vi "ADC_WRITE CONFIG.vi"(7 "Espera acceso USB":u32, 8 "error in 2":errorcluster, 10 "Dac Data IN":u16, 11 "ftHandle_in 2":u32) -> (0 "error out":errorcluster, 3 "ftHandle_out":u32)   [LabVIEW 2019]
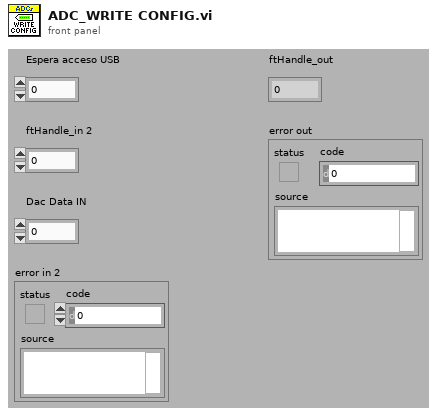
[diagram p1: front panel]
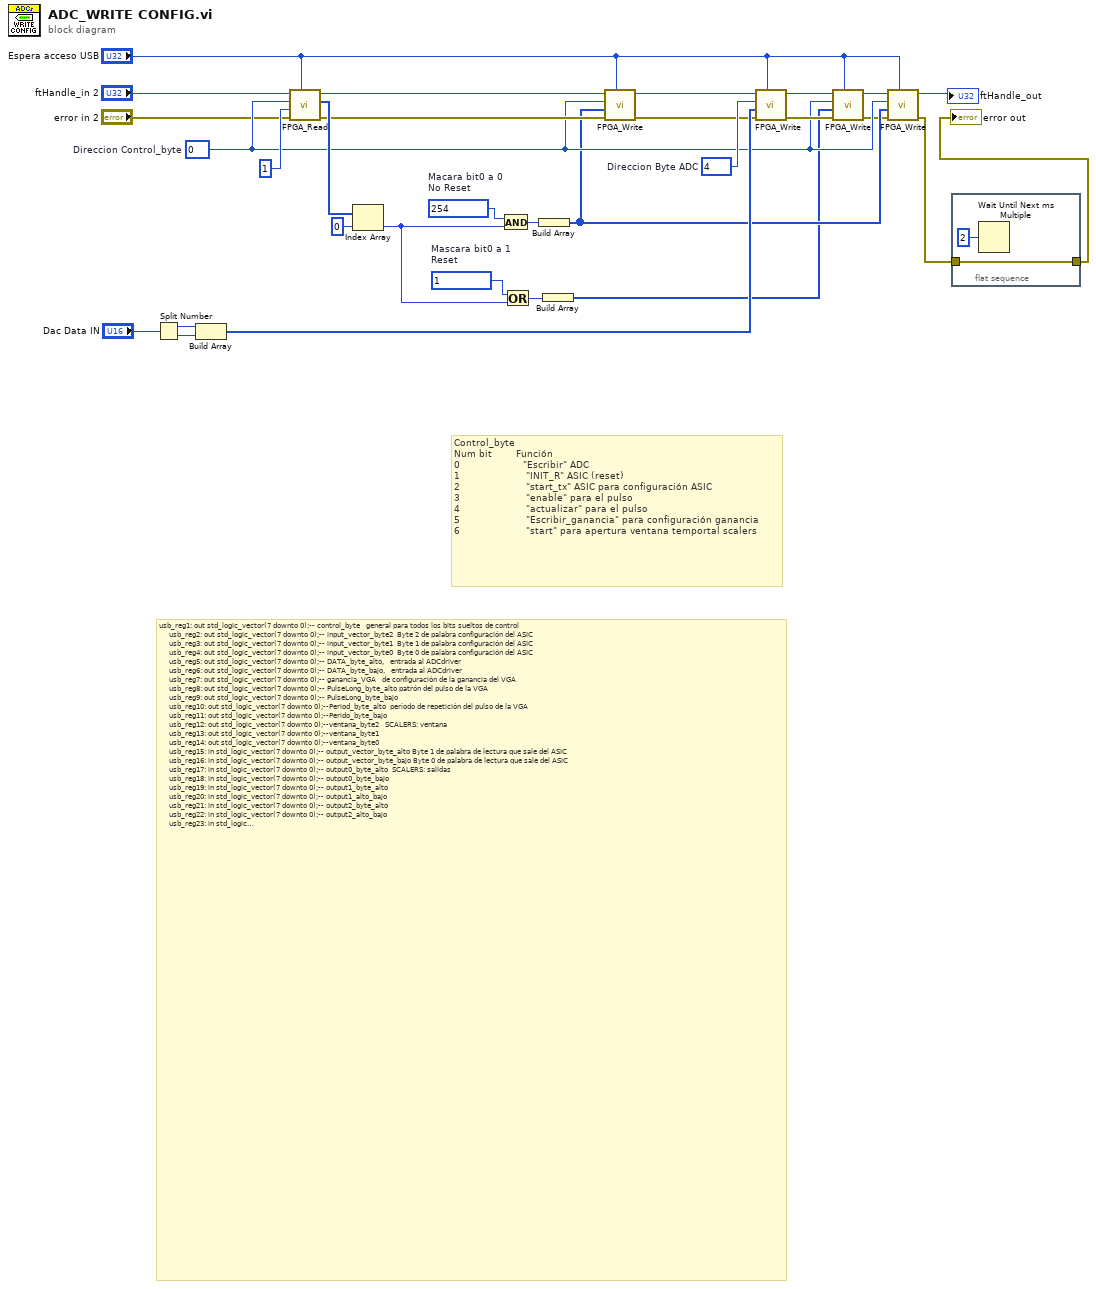
[diagram p0: block diagram]
diagram:
  w26 = u8 4  # Direccion Byte ADC
  w20 = u8 1  # Mascara bit0 a 1 Reset
  w18 = u8 254  # Macara bit0 a 0 No Reset
  w10 = u8 0  # Direccion Control_byte
  # "Control_byte\nNum bit        Función\n0                     \"Escribir\" ADC\n1                      \"INIT_R\" ASIC (reset)\n2                      \"start_tx\" ASIC para configuración ASIC\n3                      \"enable\" para el pulso\n4                      \"actualizar\" para el pulso\n5                      \"Escribir_ganancia\" para configuración ganancia\n6                      \"start\" para apertura ventana temportal scalers"
  # "usb_reg1: out std_logic_vector(7 downto 0);-- control_byte\t\t\tgeneral para todos los bits sueltos de control\n\t\t\t  usb_reg2: out std_logic_vector(7 downto 0);-- input_vector_byte2 \tByte 2 de palabra configuración del ASIC\n\t\t\t  usb_reg3: out std_logic_vector(7 downto 0);-- input_vector_byte1 \tByte 1 de palabra configuración del ASIC\n\t\t\t  usb_reg4: out std_logic_vector(7 downto 0);-- input_vector_byte0 \tByte 0 de palabra configuración del ASIC\n\t\t\t  usb_reg5: out std_logic_vector(7 downto 0);-- DATA_byte_alto, \t\tentrada al ADCdriver\n\t\t\t  usb_reg6: out std_logic_vector(7 downto 0);-- DATA_byte_bajo, \t\tentrada al ADCdriver\n\t\t\t  usb_reg7: out std_logic_vector(7 downto 0);-- ganancia_VGA\t\t\tde configuración de la ganancia del VGA\n\t\t\t  usb_reg8: out std_logic_vector(7 downto 0);-- PulseLong_byte_alto\tpatrón del pulso de la VGA\n\t\t\t  usb_reg9: out std_logic_vector(7 downto 0);-- PulseLong_byte_bajo\n\t\t\t  usb_reg10: out std_logic_vector(7 downto 0);--Period_byte_alto\t\tperíodo de repetición del pulso de la VGA\n\t\t\t  usb_reg11: out std_logic_vector(7 downto 0);--Perido_byte_bajo\n\t\t\t  usb_reg12: out std_logic_vector(7 downto 0);--ventana_byte2\t\t\tSCALERS: ventana\n\t\t\t  usb_reg13: out std_logic_vector(7 downto 0);--ventana_byte1\t\n\t\t\t  usb_reg14: out std_logic_vector(7 downto 0);--ventana_byte0\n\t\t\t  usb_reg15: in std_logic_vector(7 downto 0);-- output_vector_byte_alto\tByte 1 de palabra de lectura que sale del ASIC\n\t\t\t  usb_reg16: in std_logic_vector(7 downto 0);-- output_vector_byte_bajo\tByte 0 de palabra de lectura que sale del ASIC\n\t\t\t  usb_reg17: in std_logic_vector(7 downto 0);-- output0_byte_alto\t\tSCALERS: salidas\n\t\t\t  usb_reg18: in std_logic_vector(7 downto 0);-- output0_byte_bajo\n\t\t\t  usb_reg19: in std_logic_vector(7 downto 0);-- output1_byte_alto\n\t\t\t  usb_reg20: in std_logic_vector(7 downto 0);-- output1_alto_bajo \n\t\t\t  usb_reg21: in std_logic_vector(7 downto 0);-- output2_byte_alto \n\t\t\t  usb_reg22: in std_logic_vector(7 downto 0);-- output2_alto_bajo \n\t\t\t  usb_reg23: in std_logic_vector(7 downto 0);-- para el canal_0 del ADCdriver\n\t\t\t  usb_reg24: in std_logic_vector(7 downto 0);\n\t\t\t  usb_reg25: in std_logic_vector(7 downto 0);-- para el canal_1 del ADCdriver\n\t\t\t  usb_reg26: in std_logic_vector(7 downto 0);\n\t\t\t  usb_reg27: in std_logic_vector(7 downto 0);-- para el canal_2 del ADCdriver\n\t\t\t  usb_reg28: in std_logic_vector(7 downto 0);\n\t\t\t  usb_reg29: in std_logic_vector(7 downto 0);-- para el canal_3 del ADCdriver\n\t\t\t  usb_reg30: in std_logic_vector(7 downto 0);\n\t\t\t  usb_reg31: in std_logic_vector(7 downto 0);-- para el canal_4 del ADCdriver\n\t\t\t  usb_reg32: in std_logic_vector(7 downto 0);\n\t\t\t  usb_reg33: in std_logic_vector(7 downto 0);-- para el canal_5 del ADCdriver\n\t\t\t  usb_reg34: in std_logic_vector(7 downto 0);\n\t\t\t  usb_reg35: in std_logic_vector(7 downto 0);-- para el canal_6 del ADCdriver\n\t\t\t  usb_reg36: in std_logic_vector(7 downto 0);\n\t\t\t  usb_reg37: in std_logic_vector(7 downto 0);-- para el canal_7 del ADCdriver\n\t\t\t  usb_reg38: in std_logic_vector(7 downto 0);\n\t\t\t  usb_reg39: in std_logic_vector(7 downto 0);-- para el canal_8 del ADCdriver\n\t\t\t  usb_reg40: in std_logic_vector(7 downto 0);\n\t\t\t  usb_reg41: in std_logic_vector(7 downto 0);-- para el canal_9 del ADCdriver\n\t\t\t  usb_reg42: in std_logic_vector(7 downto 0);\n\t\t\t  usb_reg43: in std_logic_vector(7 downto 0);-- para el canal_10 del ADCdriver\n\t\t\t  usb_reg44: in std_logic_vector(7 downto 0)--;"
  n1 = Split Number(x="Dac Data IN") -> (hi(x)=w28:u8, lo(x)=w29:u8)
  n2 = Build Array(w28, w29) -> (w30:u8[])
  n3 = call "FPGA_Read.vi"("Espera acceso USB"="Espera acceso USB", "error in"="error in 2", "Numero Bytes"=u8 1, "Dirección base"=w10, "ftHandle_in"="ftHandle_in 2") -> ("error out"=w13:errorcluster, "lpBuffer_out"=w14:u8[], "ftHandle_out"=w12:u32)  [unwired: 2 in, 2 out]
  n4 = Index Array(array=w14, index=0) -> (element=w19:u8)
  n5 = And(x=w18, y=w19) -> (x .and. y?=w16:u8)
  n6 = Or(x=w20, y=w19) -> (x .or. y?=w17:u8)
  n7 = Build Array(w16) -> (w6:u8[])
  n8 = Build Array(w17) -> (w3:u8[])
  n9 = call "FPGA_Write.vi"("Espera acceso USB"="Espera acceso USB", "error in"=w13, "Bytes de escritura"=w6, "Dirección base"=w10, "ftHandle_in"=w12) -> ("error out"=w22:errorcluster, "ftHandle_out"=w21:u32)  [unwired: 1 in, 2 out]
  n10 = call "FPGA_Write.vi"("Espera acceso USB"="Espera acceso USB", "error in"=w22, "Bytes de escritura"=w30, "Dirección base"=w26, "ftHandle_in"=w21) -> ("error out"=w25:errorcluster, "ftHandle_out"=w24:u32)  [unwired: 1 in, 2 out]
  n11 = call "FPGA_Write.vi"("Espera acceso USB"="Espera acceso USB", "error in"=w25, "Bytes de escritura"=w3, "Dirección base"=w10, "ftHandle_in"=w24) -> ("error out"=w4:errorcluster, "ftHandle_out"=w5:u32)  [unwired: 1 in, 2 out]
  n12 = call "FPGA_Write.vi"("Espera acceso USB"="Espera acceso USB", "error in"=w4, "Bytes de escritura"=w6, "Dirección base"=w10, "ftHandle_in"=w5) -> ("error out"=w2:errorcluster, "ftHandle_out"=→"ftHandle_out":u32)  [unwired: 1 in, 2 out]
  n13 = flat-sequence {
    tunnel: w2 -> [w31]
    tunnel: [w31] -> w1
    frame #0 {
      n14 = Wait Until Next ms Multiple(millisecond multiple=u32 2) -> ()  [unwired: 1 out]
    }
  }
  "error out" <- w1
